vi "AuMT8852B Tester Identity.vi"(8 "error in (no error)":errorcluster, 11 "VISA session":refnum<visa-resource-name>) -> (0 "error out":errorcluster, 2 "error code":i32, 3 "VISA session out":refnum<visa-resource-name>, 4 "Tester Identity":T1)   [LabVIEW 2017]
doc: "Anritsu MT8852B Bluetooth Tester\n\nObtains the identity, serial number and firmware version number of the Anritsu Bluetooth test set. The response is the same as the standard *IDN? command and displays the following:\n\nManufacturer's name\nModel number\nSerial number\nSoftware revision"
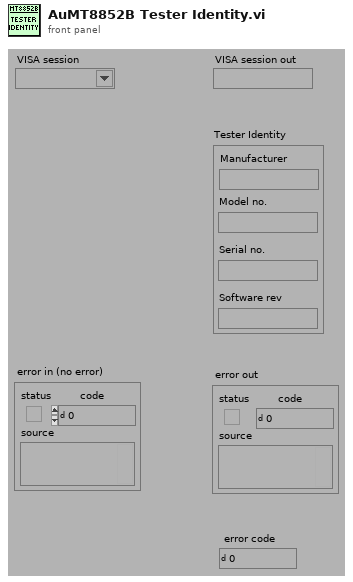
[diagram p1: front panel]
types:
  T1 = cluster{"Manufacturer":string, "Model no.":string, "Software rev":string, "Serial no.":string}
  T2 = enum16{"Simulate", "Range check", "Cache", "Query instrument status"}
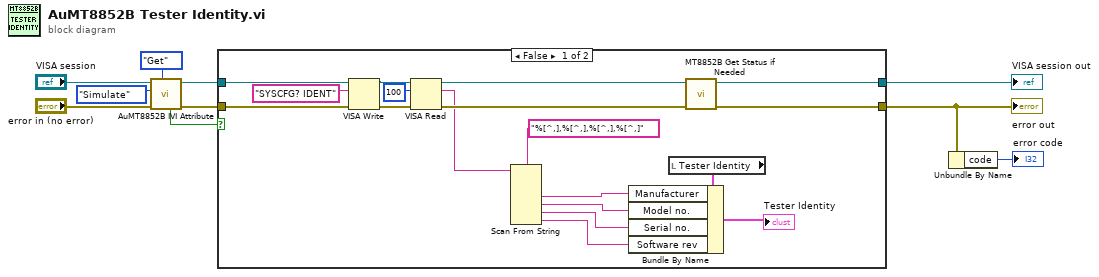
[diagram p0: block diagram]
diagram:
  n1 = call <instrlib>:"AuMT8852B IVI Attribute.vi"("Set/Get (Set)"=enum16{"Set", "Get"}."Get", "error in (no error)"="error in (no error)", "Flag (Simulate)"=T2."Simulate", "VISA session"="VISA session") -> ("error out"=w7:errorcluster, "VISA session out"=w9:refnum<visa-resource-name>, "Value out"=w3:bool)  [unwired: 5 in]
  n2 = case shown="False" w3 {
    tunnel: [w20 w30] -> w10
    tunnel: [w19 w29] -> w1
    tunnel: w9 -> [w27 w30]
    tunnel: w7 -> [w26 w29]
    frame False {
      n3 = VISA Write(VISA resource name=w27, write buffer="SYSCFG? IDENT" ("write buffer (\"\")"), error in (no error)=w26) -> (VISA resource name out=w25:refnum<visa-resource-name>, error out=w24:errorcluster)  [unwired: 1 out]
      n4 = VISA Read(VISA resource name=w25, byte count=u32 100 ("byte count (0)"), error in (no error)=w24) -> (VISA resource name out=w17:refnum<visa-resource-name>, read buffer=w15:string, error out=w18:errorcluster)  [unwired: 1 out]
      n5 = Scan From String(format string="%[^,],%[^,],%[^,],%[^,]" ("write buffer (\"\")"), input string=w15) -> (output 1=w14:string, output 2=w11:string, output 3=w13:string, output 4=w12:string)  [unwired: 6 in, 3 out]
      n6 = local read "Tester Identity"() -> (w22:T1)
      n7 = Bundle By Name(cluster=w22, "Manufacturer"=w14, "Model no."=w11, "Serial no."=w13, "Software rev"=w12) -> (→"Tester Identity":T1)
      n8 = call <instrlib>:"MT8852B Get Status if Needed.vi"("error in (no error)"=w18, "VISA session"=w17) -> ("error out"=w19:errorcluster, "VISA session out"=w20:refnum<visa-resource-name>)  [unwired: 8 in]
    }
    frame True {
    }
  }
  "error out" <- w1
  "VISA session out" <- w10
  n9 = Unbundle By Name(w1) -> ("code"=→"error code":i32)
